vi "SHsUmrechnen-01-17.vi"(6 "TemperaturenSH[V]":dbl[](array[numeric]), 7 "SpannungenSH[V]":dbl[](array[numeric]), 9 "Traps/MachKoeff2":dbl[](array[numeric]), 10 "Traps/MachKoeff1":dbl[](array[numeric]), 11 "Traps/MachKoeff0":dbl[](array[numeric])) -> (2 "Spannungen SH":T1 {"USetp [V]Mach1" format="%.12g"; "[1]" format="%.14g"; "[2]" format="%.14g"; "[3]" format="%.14g"; "[4]" format="%.14g"; "[5]" format="%.14g"; "[6]" format="%.14g"; "[7]" format="%.14g"; "[8]" format="%.14g"}, 3 "TemperaturenSH[°C]":dbl[](array[numeric]))   [LabVIEW 2010]
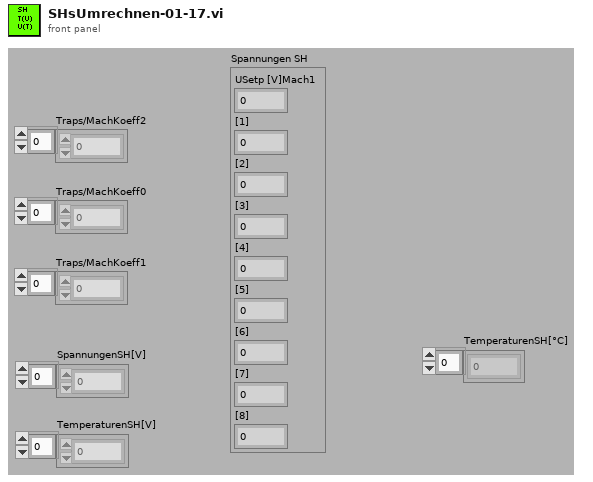
[diagram p1: front panel]
types:
  T1 = cluster{"USetp [V]Mach1":fxp<+/-,16,6>, "[1]":fxp<+/-,16,4>, "[2]":fxp<+/-,16,4>, "[3]":fxp<+/-,16,4>, "[4]":fxp<+/-,16,4>, "[5]":fxp<+/-,16,4>, "[6]":fxp<+/-,16,4>, "[7]":fxp<+/-,16,4>, "[8]":fxp<+/-,16,4>}
  T2 = cluster{"[0]":fxp<+/-,16,4>, "[1]":fxp<+/-,16,4>, "[2]":fxp<+/-,16,4>, "[3]":fxp<+/-,16,4>, "[4]":fxp<+/-,16,4>, "[5]":fxp<+/-,16,4>, "[6]":fxp<+/-,16,4>, "[7]":fxp<+/-,16,4>, "[8]":fxp<+/-,16,4>}
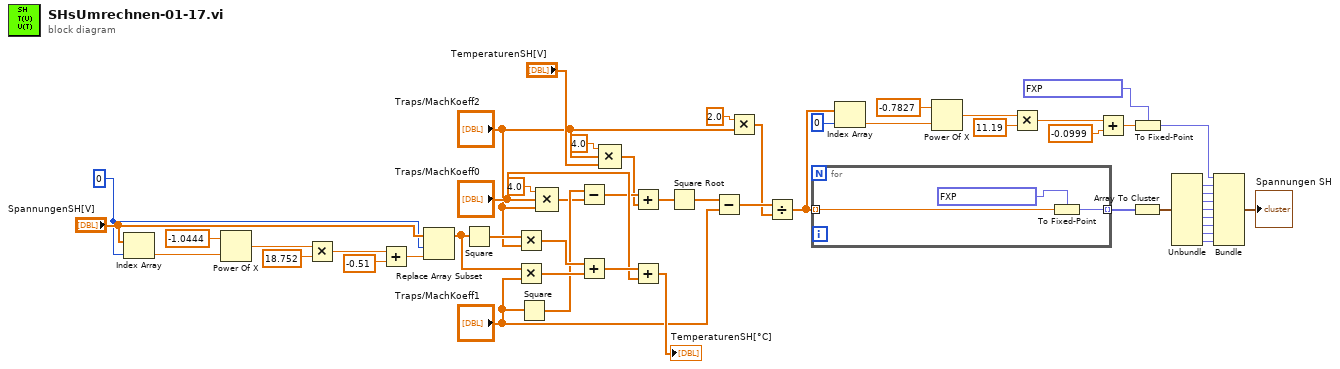
[diagram p0: block diagram]
diagram:
  w3 = 0 ("index")
  n1 = Index Array(array="SpannungenSH[V]", index=w3) -> (element=w5:dbl)
  n2 = Power Of X(1:w5, 2:-1.0444 ("x")) -> (0:w10:dbl)
  n3 = Multiply(x=w10, y=18.752) -> (x*y=w8:dbl)
  n4 = Add(x=w8, y=-0.51) -> (x+y=w2:dbl)
  n5 = Replace Array Subset(array="SpannungenSH[V]", new element=w2, index=w3) -> (w1:dbl[])
  n6 = Square(x=w1) -> (x^2=w49:dbl[])
  n7 = Multiply(x=w49, y="Traps/MachKoeff2") -> (x*y=w50:dbl[])
  n8 = Multiply(x=w1, y="Traps/MachKoeff1") -> (x*y=w51:dbl[])
  n9 = Square(x="Traps/MachKoeff1") -> (x^2=w43:dbl[])
  n10 = Compound Arithmetic op=MULTIPLY(4.0, "Traps/MachKoeff0", "Traps/MachKoeff2") -> (w42:dbl[])
  n11 = Subtract(x=w43, y=w42) -> (x-y=w41:dbl[])
  n12 = Add(x=w50, y=w51) -> (x+y=w52:dbl[])
  n13 = Compound Arithmetic op=MULTIPLY(4.0, "Traps/MachKoeff2", "TemperaturenSH[V]") -> (w40:dbl[])
  n14 = Add(x=w41, y=w40) -> (x+y=w39:dbl[])
  n15 = Add(x=w52, y="Traps/MachKoeff0") -> (x+y=→"TemperaturenSH[°C]":dbl[])
  n16 = Square Root(x=w39) -> (sqrt(x)=w38:dbl[])
  n17 = Subtract(x=w38, y="Traps/MachKoeff1") -> (x-y=w36:dbl[])
  n18 = Multiply(x=2.0, y="Traps/MachKoeff2") -> (x*y=w33:dbl[])
  n19 = Divide(x=w36, y=w33) -> (x/y=w26:dbl[])
  n20 = for {
    tunnel: w26 -> [w55] mode=indexing
    tunnel: [w54] -> w24 mode=indexing
    n21 = To Fixed-Point(fixed-point type=fxp<+/-,16,4> 0.0 ("USetp [V]Mach1"), number=w55) -> (fixed-point=w54:fxp<+/-,16,4>)
  }
  n22 = Index Array(array=w26, index=0) -> (element=w28:dbl)
  n23 = Power Of X(1:w28, 2:-0.7827 ("y")) -> (0:w32:dbl)
  n24 = Multiply(x=w32, y=11.19) -> (x*y=w30:dbl)
  n25 = Add(x=w30, y=-0.0999) -> (x+y=w23:dbl)
  n26 = Array To Cluster(array=w24) -> (cluster=w21:T2)
  n27 = To Fixed-Point(fixed-point type=fxp<+/-,16,6> 0.0 ("USetp [V]Mach1"), number=w23) -> (fixed-point=w12:fxp<+/-,16,6>)
  n28 = Unbundle(w21) -> ("[1]"=w20:fxp<+/-,16,4>, "[2]"=w19:fxp<+/-,16,4>, "[3]"=w18:fxp<+/-,16,4>, "[4]"=w17:fxp<+/-,16,4>, "[5]"=w16:fxp<+/-,16,4>, "[6]"=w15:fxp<+/-,16,4>, "[7]"=w14:fxp<+/-,16,4>, "[8]"=w13:fxp<+/-,16,4>)  [unwired: 1 out]
  n29 = Bundle("USetp [V]Mach1"=w12, "[1]"=w20, "[2]"=w19, "[3]"=w18, "[4]"=w17, "[5]"=w16, "[6]"=w15, "[7]"=w14, "[8]"=w13) -> (→"Spannungen SH":T1)  [unwired: 1 in]
